vi "TagBus_Initialize_Merge Tags.vi"(8 "error in (no error)":errorcluster, 10 "Current TagDescriptions":refnum<class "tag descriptor.lvclass">[](array[class]), 11 "New TagDescriptions":refnum<class "tag descriptor.lvclass">[](array[class])) -> (0 "error out":errorcluster, 3 "TagDescriptions":refnum<class "tag descriptor.lvclass">[](array[class]))   [LabVIEW 2015, in "TagBus.lvclass"]
uses:
  TagBus.lvclass
  <vilib>/NI/Tag Bus/tag/tag descriptor.lvclass
  <vilib>/NI/Tag Bus/tag/tag descriptor.lvclass/tag descriptor.ctl
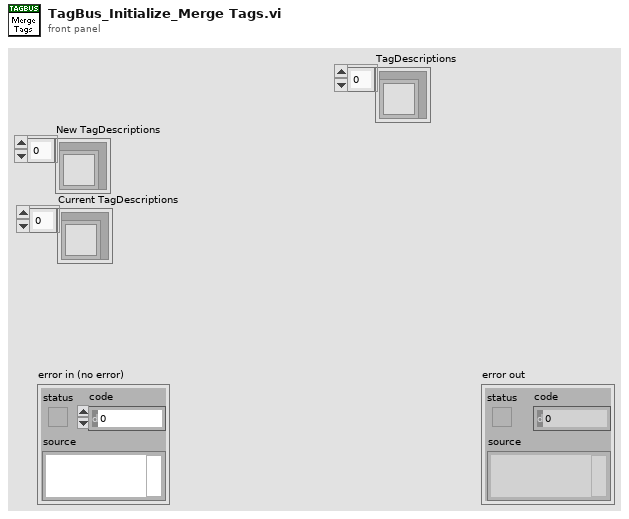
[diagram p1: front panel]
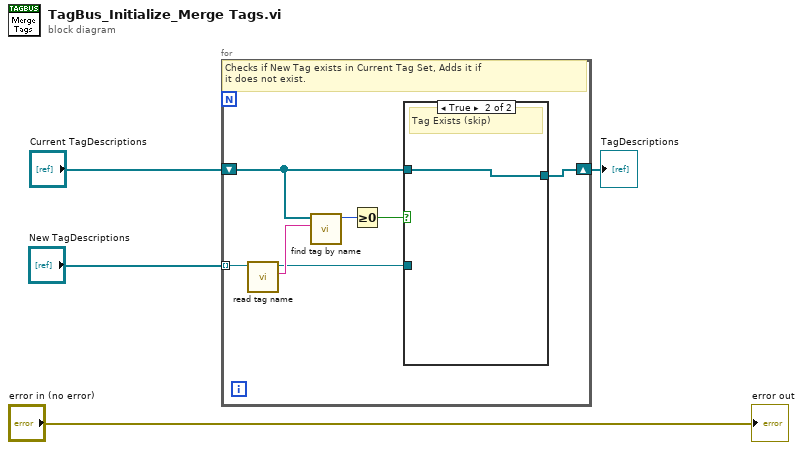
[diagram p0: block diagram]
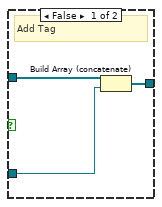
[diagram p2: hidden frame]
diagram:
  n1 = for {
    tunnel: "New TagDescriptions" -> [w11] mode=indexing
    shift-right: [w6] -> w1
    shift-left: "Current TagDescriptions" -> [w8]
    # "Checks if New Tag exists in Current Tag Set, Adds it if\nit does not exist."
    n2 = call <vilib>:"read tag name.vi"("system tag in"=w11) -> ("name"=w10:string, "system tag out"=w5:refnum<class "tag descriptor.lvclass">)  [unwired: 8 in, 1 out]
    n3 = call <vilib>:"find tag by name.vi"("name"=w10, "tags in"=w8) -> ("index"=w9:i32)  [unwired: 9 in]
    n4 = Greater Or Equal To 0?(x=w9) -> (x >= 0?=w7:bool)
    n5 = case shown="True" w7 {
      tunnel: w8 -> [w14 w15]
      tunnel: [w13 w15] -> w6
      tunnel: w5 -> [w12 _]
      frame False {
        # "Add Tag"
        n6 = Build Array (concatenate)(w14, w12) -> (w13:refnum<class "tag descriptor.lvclass">[])
      }
      frame True {
        # "Tag Exists (skip)"
      }
    }
  }
  "TagDescriptions" <- w1
  "error out" <- "error in (no error)"
